vi "DN4_Counter_DetectCntrEvent_Ex.vi"(4 "error in (no error)":errorcluster, 5 "status":bool, 7 "Task ID":u32) -> (0 "error out":errorcluster, 1 "interrupt?":bool, 2 "interrupt source":i32, 3 "Task out ID":u32)   [LabVIEW 2009]
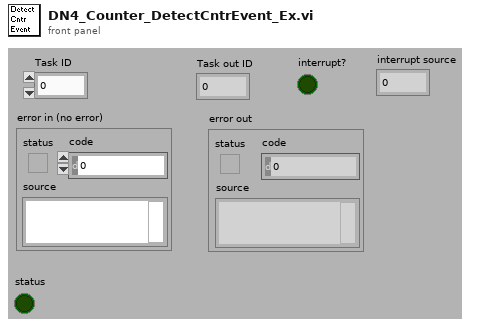
[diagram p1: front panel]
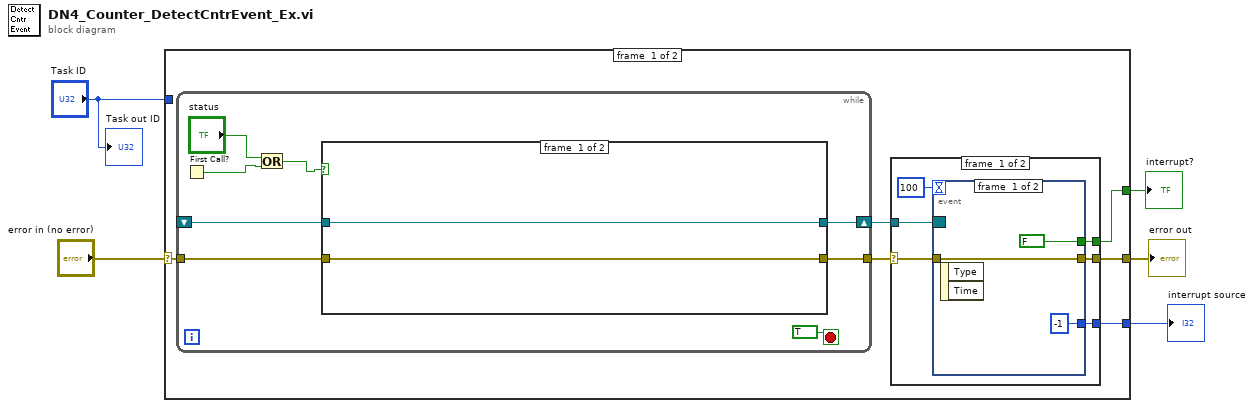
[diagram p0: block diagram]
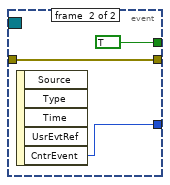
[diagram p2: hidden frame]
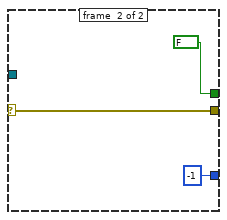
[diagram p3: hidden frame]
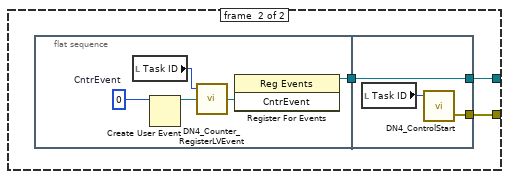
[diagram p4: hidden frame]
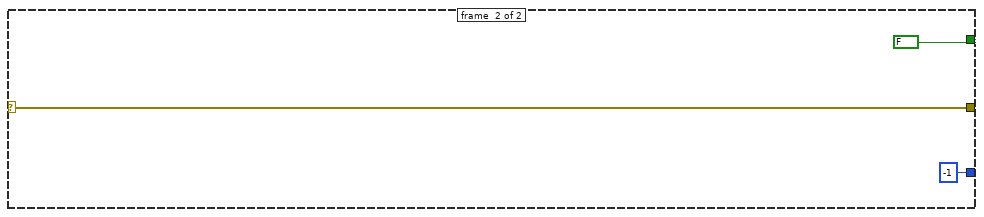
[diagram p5: hidden frame]
diagram:
  n1 = case shown="No Error" "error in (no error)" {
    selector: "error in (no error)" -> [w7 w49]
    tunnel: "Task ID" -> [_ _]
    tunnel: [w11 FALSE] -> w4
    tunnel: [w10 w49] -> w3
    tunnel: [w6 -1 ("CntrEvent")] -> w1
    frame #0 {
      n2 = while {
        shift-right: [w33] -> w9
        shift-left: _ -> [w32]
        tunnel: [w31] -> w8
        tunnel: w7 -> [w30]
        stop <- TRUE stop-if-true
        n3 = First Call?() -> (First Call?: T/F=w28:bool)
        n4 = Or(x="status", y=w28) -> (x .or. y?=w27:bool)
        n5 = case shown="True" w27 {
          tunnel: [w36 w38] -> w33
          tunnel: w32 -> [w36 _]
          tunnel: [w35 w37] -> w31
          tunnel: w30 -> [w35 _]
          frame #0 {
          }
          frame #1 {
            n6 = flat-sequence {
              tunnel: [w40] -> w39
              tunnel: [w46] -> w38
              tunnel: w39 -> [w46]
              tunnel: [w45] -> w37
              frame #0 {
                w44 = 0  # CntrEvent
                n7 = local read "Task ID"() -> (w43:u32)
                n8 = Create User Event(user event datatype=w44) -> (user event=w42:refnum<user-event>)  [unwired: 1 in, 1 out]
                n9 = call <userlib>:"DN4_Counter_RegisterLVEvent.vi"("CntrEvent"=w42, "Task ID"=w43) -> ("CntrEvent"=w41:refnum<user-event>)  [unwired: 1 in, 2 out]
                n10 = register-events(w41) -> (reference out=w40:refnum<event-registration>)  [unwired: 2 in, 1 out]
              }
              frame #1 {
                n11 = local read "Task ID"() -> (w47:u32)
                n12 = call <userlib>:"DN4_ControlStart.vi"("Task ID"=w47) -> ("error out"=w45:errorcluster)  [unwired: 1 in, 2 out]
              }
            }
          }
        }
      }
      n13 = case shown="No Error" w8 {
        selector: w8 -> [w14 w25]
        tunnel: w9 -> [w17 _]
        tunnel: [w16 FALSE] -> w11
        tunnel: [w13 w25] -> w10
        tunnel: [w12 -1 ("CntrEvent")] -> w6
        frame #0 {
          n14 = event shown="[1] <CntrEvent>: User Event" {
            selector: w17 -> [_ _]
            dyn-events: _ -> [_ _]
            timeout: 100 -> [_ _]
            tunnel: [FALSE TRUE] -> w16
            tunnel: w14 -> [w19 w22]
            tunnel: [w19 w22] -> w13
            tunnel: [-1 ("CntrEvent") w21] -> w12
            event #0 {
              n15 = event-data() -> ()  [unwired: 3 out]
            }
            event #1 {
              n16 = event-data() -> ("CntrEvent"=w21:i32)  [unwired: 5 out]
            }
          }
        }
        frame #1 {
        }
      }
    }
    frame #1 {
    }
  }
  "error out" <- w3
  "interrupt?" <- w4
  "interrupt source" <- w1
  "Task out ID" <- "Task ID"
